vi "Write Process Program CEID.vi"(8 "error in (no error)":errorcluster, 10 "Process Program CEID":u32, 11 "14-Process Program Creating Editing or Deleting in":refnum<class "14-Process Program Creating Editing or Deleting.lvclass">) -> (0 "error out":errorcluster, 3 "14-Process Program Creating Editing or Deleting out":refnum<class "14-Process Program Creating Editing or Deleting.lvclass">)   [LabVIEW 2020, in "SECS Scenarios.lvlib" / "14-Process Program Creating Editing or Deleting.lvclass"]
uses:
  14-Process Program Creating Editing or Deleting.lvclass
  14-Process Program Creating Editing or Deleting.lvclass/14-Process Program Creating Editing or Deleting.ctl
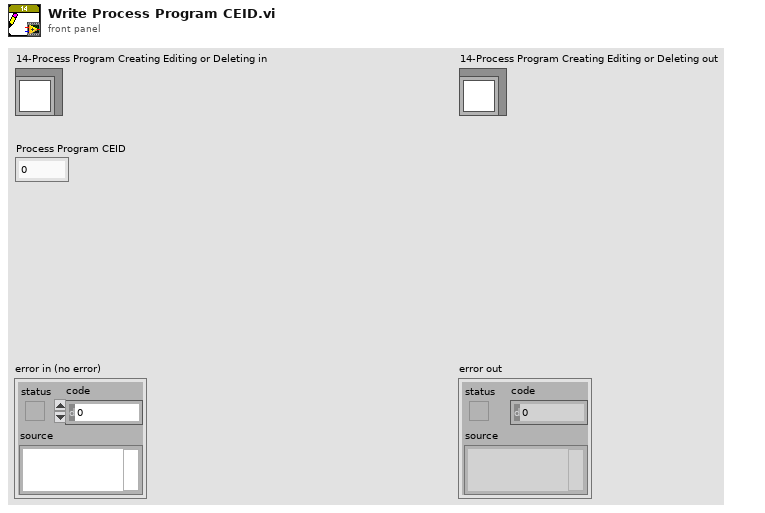
[diagram p1: front panel]
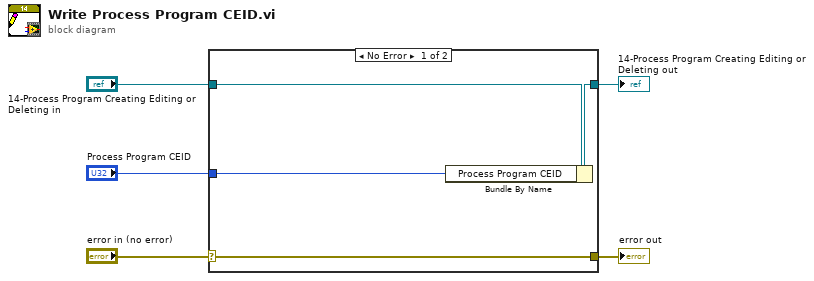
[diagram p0: block diagram]
diagram:
  n1 = case shown="No Error" "error in (no error)" {
    selector: "error in (no error)" -> [w9 w10]
    tunnel: [w9 w10] -> w4
    tunnel: [w7 w11] -> w2
    tunnel: "14-Process Program Creating Editing or Deleting in" -> [w8 w11]
    tunnel: "Process Program CEID" -> [w6 _]
    frame No Error {
      n2 = Bundle By Name(cluster=w8, "Process Program CEID"=w6) -> (w7:refnum<class "14-Process Program Creating Editing or Deleting.lvclass">)
    }
    frame Error {
    }
  }
  "error out" <- w4
  "14-Process Program Creating Editing or Deleting out" <- w2
